vi "MotionProfileUpdateBuffers.vi"(3 "error in":errorcluster, 4 "RobotConfig":T1={"Motors"={"DriveRightPrimary"={"CAN Address"=3, "Invert"=FALSE, "InvertSensor"=FALSE, "Unit Conversion Factor"=0.0, "Brake Mode"=enum."Override to Brake", "Reverse Limt Switch Mode"=enum."Normally Closed", "Forward Limt Swith Mode"=enum."Normally Closed", "PWM Channel"=enum."Invalid", "Motor Controller Type"=enum."Talon SRX", "Peak Current (A)"=0, "Continuos Current (A)"=0, "Peak Duration (ms)"=0, "Current Limit Enable"=FALSE}, "DriveRightSecondary"={"CAN Address"=2, "Invert"=FALSE, "InvertSensor"=FALSE, "Unit Conversion Factor"=0.0, "Brake Mode"=enum."Override to Brake", "Reverse Limt Switch Mode"=enum."Normally Closed", "Forward Limt Swith Mode"=enum."Normally Closed", "PWM Channel"=enum."Invalid", "Motor Controller Type"=enum."Talon SRX", "Peak Current (A)"=0, "Continuos Current (A)"=0, "Peak Duration (ms)"=0, "Current Limit Enable"=FALSE}, "DriveLeftPrimary"={"CAN Address"=1, "Invert"=FALSE, "InvertSensor"=FALSE, "Unit Conversion Factor"=0.0, "Brake Mode"=enum."Override to Brake", "Reverse Limt Switch Mode"=enum."Normally Closed", "Forward Limt Swith Mode"=enum."Normally Closed", "PWM Channel"=enum."Invalid", "Motor Controller Type"=enum."Talon SRX", "Peak Current (A)"=0, "Continuos Current (A)"=0, "Peak Duration (ms)"=0, "Current Limit Enable"=FALSE}, "DriveLeftSecondary"={"CAN Address"=4, "Invert"=FALSE, "InvertSensor"=FALSE, "Unit Conversion Factor"=0.0, "Brake Mode"=enum."Override to Brake", "Reverse Limt Switch Mode"=enum."Normally Closed", "Forward Limt Swith Mode"=enum."Normally Closed", "PWM Channel"=enum."Invalid", "Motor Controller Type"=enum."Talon SRX", "Peak Current (A)"=0, "Continuos Current (A)"=0, "Peak Duration (ms)"=0, "Current Limit Enable"=FALSE}, "RearClimb"={"CAN Address"=8, "Invert"=FALSE, "InvertSensor"=FALSE, "Unit Conversion Factor"=0.0, "Brake Mode"=enum."Override to Brake", "Reverse Limt Switch Mode"=enum."Normally Closed", "Forward Limt Swith Mode"=enum."Normally Closed", "PWM Channel"=enum."Invalid", "Motor Controller Type"=enum."Talon SRX", "Peak Current (A)"=0, "Continuos Current (A)"=0, "Peak Duration (ms)"=0, "Current Limit Enable"=FALSE}, "Front Climb"={"CAN Address"=7, "Invert"=FALSE, "InvertSensor"=FALSE, "Unit Conversion Factor"=0.0, "Brake Mode"=enum."Override to Brake", "Reverse Limt Switch Mode"=enum."Normally Closed", "Forward Limt Swith Mode"=enum."Normally Closed", "PWM Channel"=enum."Invalid", "Motor Controller Type"=enum."Talon SRX", "Peak Current (A)"=0, "Continuos Current (A)"=0, "Peak Duration (ms)"=0, "Current Limit Enable"=FALSE}, "Climb Drive"={"CAN Address"=5, "Invert"=FALSE, "InvertSensor"=FALSE, "Unit Conversion Factor"=0.0, "Brake Mode"=enum."Override to Brake", "Reverse Limt Switch Mode"=enum."Normally Closed", "Forward Limt Swith Mode"=enum."Normally Closed", "PWM Channel"=enum."Invalid", "Motor Controller Type"=enum."Talon SRX", "Peak Current (A)"=0, "Continuos Current (A)"=0, "Peak Duration (ms)"=0, "Current Limit Enable"=FALSE}, "Shoulder1"={"CAN Address"=6, "Invert"=FALSE, "InvertSensor"=FALSE, "Unit Conversion Factor"=0.0, "Brake Mode"=enum."Override to Brake", "Reverse Limt Switch Mode"=enum."Normally Closed", "Forward Limt Swith Mode"=enum."Normally Closed", "PWM Channel"=enum."Invalid", "Motor Controller Type"=enum."Talon SRX", "Peak Current (A)"=0, "Continuos Current (A)"=0, "Peak Duration (ms)"=0, "Current Limit Enable"=FALSE}, "Shoulder2"={"CAN Address"=9, "Invert"=FALSE, "InvertSensor"=FALSE, "Unit Conversion Factor"=0.0, "Brake Mode"=enum."Override to Brake", "Reverse Limt Switch Mode"=enum."Normally Closed", "Forward Limt Swith Mode"=enum."Normally Closed", "PWM Channel"=enum."Invalid", "Motor Controller Type"=enum."Talon SRX", "Peak Current (A)"=0, "Continuos Current (A)"=0, "Peak Duration (ms)"=0, "Current Limit Enable"=FALSE}, "Wrist"={"CAN Address"=10, "Invert"=FALSE, "InvertSensor"=FALSE, "Unit Conversion Factor"=0.0, "Brake Mode"=enum."Override to Brake", "Reverse Limt Switch Mode"=enum."Disabled", "Forward Limt Swith Mode"=enum."Disabled", "PWM Channel"=enum."Invalid", "Motor Controller Type"=enum."Talon SRX", "Peak Current (A)"=0, "Continuos Current (A)"=0, "Peak Duration (ms)"=0, "Current Limit Enable"=FALSE}, "Extension"={"CAN Address"=11, "Invert"=FALSE, "InvertSensor"=FALSE, "Unit Conversion Factor"=0.0, "Brake Mode"=enum."Override to Brake", "Reverse Limt Switch Mode"=enum."Disabled", "Forward Limt Swith Mode"=enum."Disabled", "PWM Channel"=enum."Invalid", "Motor Controller Type"=enum."Talon SRX", "Peak Current (A)"=0, "Continuos Current (A)"=0, "Peak Duration (ms)"=0, "Current Limit Enable"=FALSE}, "Intake1"={"CAN Address"=0, "Invert"=FALSE, "InvertSensor"=FALSE, "Unit Conversion Factor"=1.0, "Brake Mode"=enum."Override to Brake", "Reverse Limt Switch Mode"=enum."Disabled", "Forward Limt Swith Mode"=enum."Normally Open", "PWM Channel"=enum."PWM 8", "Motor Controller Type"=enum."Talon SR", "Peak Current (A)"=0, "Continuos Current (A)"=0, "Peak Duration (ms)"=0, "Current Limit Enable"=FALSE}, "Intake2"={"CAN Address"=10, "Invert"=FALSE, "InvertSensor"=TRUE, "Unit Conversion Factor"=0.0, "Brake Mode"=enum."Override to Brake", "Reverse Limt Switch Mode"=enum."Normally Open", "Forward Limt Swith Mode"=enum."Normally Open", "PWM Channel"=enum."PWM 0", "Motor Controller Type"=enum."Disabled", "Peak Current (A)"=0, "Continuos Current (A)"=0, "Peak Duration (ms)"=0, "Current Limit Enable"=FALSE}}, "Sensors"={"IMU"={"Yaw Axis"=enum."Z", "SPI Bus"=enum."SPI MXP", "AHRS Algorithm"=enum."Complementary", "Calibration Time (s)"=3.0, "Calibrate On Open"=TRUE}}, "PID"={"FrontClimb"={"P"=0.0, "I"=0.0, "D"=0.0, "F"=0.0, "IZone"=0.0}, "RearClimb"={"P"=0.0, "I"=0.0, "D"=0.0, "F"=0.0, "IZone"=0.0}, "ArmShoulder"={"P"=0.0, "I"=0.0, "D"=0.0, "F"=0.0, "IZone"=0.0}, "ArmExtend"={"P"=0.0, "I"=0.0, "D"=0.0, "F"=0.0, "IZone"=0.0}, "ArmWrist"={"P"=0.0, "I"=0.0, "D"=0.0, "F"=0.0, "IZone"=0.0}}, "Solenoids"={" Shifter"={"SolenoidChannel"=enum."Solenoid 3", "Invert"=FALSE}, "Hatch Grip"={"SolenoidChannel"=enum."Solenoid 0", "Invert"=FALSE}, "Hatch Extend"={"SolenoidChannel"=enum."Solenoid 1", "Invert"=FALSE}, "Manipulator Slide"={"SolenoidChannel"=enum."Solenoid 2", "Invert"=FALSE}, "Hatch Floor Intake"={"SolenoidChannel"=enum."Solenoid 0", "Invert"=FALSE}}, "Enable Compressor"=TRUE, "MotionMagic"={"FrontClimb"={"CruiseVelocity"=0, "Acceleration"=0}, "RearClimb"={"CruiseVelocity"=0, "Acceleration"=0}}, "RobotDimensions"={"Length (in)"=0.0, "Shoulder Height (in)"=0.0, "Frame Height (in)"=0.0, "Arm Center to Front of Robot (in)"=0.0, "Arm Min Extension (in)"=0.0, "Arm Max Extension (in)"=0.0}, "Arm Home Position"={"Radius (in)"=0.0, "ShoulderAngle (rad)"=0.0, "WristAngle (rad)"=0.0}}, 5 "RobotMotors":T15={"DriveRightPrimary"={"DeviceStatus"={"status"=FALSE, "code"=0, "source"=""}, "Type"=enum."PWM", "PWM"={"PWM Channel"=enum."PWM 1", "DeadBand"={"Name"="", "maxPositivePwm"=0, "minPositivePwm"=0, "centerPwm"=0, "maxNegativePwm"=0, "minNegativePwm"=0, "angularRange"=0}}, "CAN"={"Device Number"=0, "SetOutput VI Ref"=variant(enum8{"Percent VBus", "Current", "Speed", "Position", "Voltage"} enum."Percent VBus"), "GetOutput VI Ref"=variant(refnum<k1> refnum), "Enable VI Ref"=variant(dbl 12.0), "Disable VI Ref"=variant(enum8{"Percent VBus", "Speed", "Position", "Slave", "Unchanged / Invalid", "Voltage Compensation", "Current", "Motion Profile"} enum."Percent VBus"), "Data"=variant}, "Invert"=FALSE, "DIO PWM"={"PWM \"Enable\" Channel"=enum."Invalid", "DIOChannel"=enum."Invalid", "PWM Rate"=0.0}}, "DriveRightSecondary"={"DeviceStatus"={"status"=FALSE, "code"=0, "source"=""}, "Type"=enum."PWM", "PWM"={"PWM Channel"=enum."PWM 1", "DeadBand"={"Name"="", "maxPositivePwm"=0, "minPositivePwm"=0, "centerPwm"=0, "maxNegativePwm"=0, "minNegativePwm"=0, "angularRange"=0}}, "CAN"={"Device Number"=0, "SetOutput VI Ref"=variant(enum8{"Percent VBus", "Current", "Speed", "Position", "Voltage"} enum."Percent VBus"), "GetOutput VI Ref"=variant(refnum<k1> refnum), "Enable VI Ref"=variant(dbl 12.0), "Disable VI Ref"=variant(enum8{"Percent VBus", "Speed", "Position", "Slave", "Unchanged / Invalid", "Voltage Compensation", "Current", "Motion Profile"} enum."Percent VBus"), "Data"=variant}, "Invert"=FALSE, "DIO PWM"={"PWM \"Enable\" Channel"=enum."Invalid", "DIOChannel"=enum."Invalid", "PWM Rate"=0.0}}, "DriveLeftPrimary"={"DeviceStatus"={"status"=FALSE, "code"=0, "source"=""}, "Type"=enum."PWM", "PWM"={"PWM Channel"=enum."PWM 1", "DeadBand"={"Name"="", "maxPositivePwm"=0, "minPositivePwm"=0, "centerPwm"=0, "maxNegativePwm"=0, "minNegativePwm"=0, "angularRange"=0}}, "CAN"={"Device Number"=0, "SetOutput VI Ref"=variant(enum8{"Percent VBus", "Current", "Speed", "Position", "Voltage"} enum."Percent VBus"), "GetOutput VI Ref"=variant(refnum<k1> refnum), "Enable VI Ref"=variant(dbl 12.0), "Disable VI Ref"=variant(enum8{"Percent VBus", "Speed", "Position", "Slave", "Unchanged / Invalid", "Voltage Compensation", "Current", "Motion Profile"} enum."Percent VBus"), "Data"=variant}, "Invert"=FALSE, "DIO PWM"={"PWM \"Enable\" Channel"=enum."Invalid", "DIOChannel"=enum."Invalid", "PWM Rate"=0.0}}, "DriveLeftSecondary"={"DeviceStatus"={"status"=FALSE, "code"=0, "source"=""}, "Type"=enum."PWM", "PWM"={"PWM Channel"=enum."PWM 1", "DeadBand"={"Name"="", "maxPositivePwm"=0, "minPositivePwm"=0, "centerPwm"=0, "maxNegativePwm"=0, "minNegativePwm"=0, "angularRange"=0}}, "CAN"={"Device Number"=0, "SetOutput VI Ref"=variant(enum8{"Percent VBus", "Current", "Speed", "Position", "Voltage"} enum."Percent VBus"), "GetOutput VI Ref"=variant(refnum<k1> refnum), "Enable VI Ref"=variant(dbl 12.0), "Disable VI Ref"=variant(enum8{"Percent VBus", "Speed", "Position", "Slave", "Unchanged / Invalid", "Voltage Compensation", "Current", "Motion Profile"} enum."Percent VBus"), "Data"=variant}, "Invert"=FALSE, "DIO PWM"={"PWM \"Enable\" Channel"=enum."Invalid", "DIOChannel"=enum."Invalid", "PWM Rate"=0.0}}, " RearClimb"={"DeviceStatus"={"status"=FALSE, "code"=0, "source"=""}, "Type"=enum."PWM", "PWM"={"PWM Channel"=enum."PWM 1", "DeadBand"={"Name"="", "maxPositivePwm"=0, "minPositivePwm"=0, "centerPwm"=0, "maxNegativePwm"=0, "minNegativePwm"=0, "angularRange"=0}}, "CAN"={"Device Number"=0, "SetOutput VI Ref"=variant(enum8{"Percent VBus", "Current", "Speed", "Position", "Voltage"} enum."Percent VBus"), "GetOutput VI Ref"=variant(refnum<k1> refnum), "Enable VI Ref"=variant(dbl 12.0), "Disable VI Ref"=variant(enum8{"Percent VBus", "Speed", "Position", "Slave", "Unchanged / Invalid", "Voltage Compensation", "Current", "Motion Profile"} enum."Percent VBus"), "Data"=variant}, "Invert"=FALSE, "DIO PWM"={"PWM \"Enable\" Channel"=enum."Invalid", "DIOChannel"=enum."Invalid", "PWM Rate"=0.0}}, "FrontClimb"={"DeviceStatus"={"status"=FALSE, "code"=0, "source"=""}, "Type"=enum."PWM", "PWM"={"PWM Channel"=enum."PWM 1", "DeadBand"={"Name"="", "maxPositivePwm"=0, "minPositivePwm"=0, "centerPwm"=0, "maxNegativePwm"=0, "minNegativePwm"=0, "angularRange"=0}}, "CAN"={"Device Number"=0, "SetOutput VI Ref"=variant(enum8{"Percent VBus", "Current", "Speed", "Position", "Voltage"} enum."Percent VBus"), "GetOutput VI Ref"=variant(refnum<k1> refnum), "Enable VI Ref"=variant(dbl 12.0), "Disable VI Ref"=variant(enum8{"Percent VBus", "Speed", "Position", "Slave", "Unchanged / Invalid", "Voltage Compensation", "Current", "Motion Profile"} enum."Percent VBus"), "Data"=variant}, "Invert"=FALSE, "DIO PWM"={"PWM \"Enable\" Channel"=enum."Invalid", "DIOChannel"=enum."Invalid", "PWM Rate"=0.0}}, "ClimbDrive"={"DeviceStatus"={"status"=FALSE, "code"=0, "source"=""}, "Type"=enum."PWM", "PWM"={"PWM Channel"=enum."PWM 1", "DeadBand"={"Name"="", "maxPositivePwm"=0, "minPositivePwm"=0, "centerPwm"=0, "maxNegativePwm"=0, "minNegativePwm"=0, "angularRange"=0}}, "CAN"={"Device Number"=0, "SetOutput VI Ref"=variant(enum8{"Percent VBus", "Current", "Speed", "Position", "Voltage"} enum."Percent VBus"), "GetOutput VI Ref"=variant(refnum<k1> refnum), "Enable VI Ref"=variant(dbl 12.0), "Disable VI Ref"=variant(enum8{"Percent VBus", "Speed", "Position", "Slave", "Unchanged / Invalid", "Voltage Compensation", "Current", "Motion Profile"} enum."Percent VBus"), "Data"=variant}, "Invert"=FALSE, "DIO PWM"={"PWM \"Enable\" Channel"=enum."Invalid", "DIOChannel"=enum."Invalid", "PWM Rate"=0.0}}, "Shoulder2"={"DeviceStatus"={"status"=FALSE, "code"=0, "source"=""}, "Type"=enum."PWM", "PWM"={"PWM Channel"=enum."PWM 1", "DeadBand"={"Name"="", "maxPositivePwm"=0, "minPositivePwm"=0, "centerPwm"=0, "maxNegativePwm"=0, "minNegativePwm"=0, "angularRange"=0}}, "CAN"={"Device Number"=0, "SetOutput VI Ref"=variant(enum8{"Percent VBus", "Current", "Speed", "Position", "Voltage"} enum."Percent VBus"), "GetOutput VI Ref"=variant(refnum<k1> refnum), "Enable VI Ref"=variant(dbl 12.0), "Disable VI Ref"=variant(enum8{"Percent VBus", "Speed", "Position", "Slave", "Unchanged / Invalid", "Voltage Compensation", "Current", "Motion Profile"} enum."Percent VBus"), "Data"=variant}, "Invert"=FALSE, "DIO PWM"={"PWM \"Enable\" Channel"=enum."Invalid", "DIOChannel"=enum."Invalid", "PWM Rate"=0.0}}, "Shoulder1 "={"DeviceStatus"={"status"=FALSE, "code"=0, "source"=""}, "Type"=enum."PWM", "PWM"={"PWM Channel"=enum."PWM 1", "DeadBand"={"Name"="", "maxPositivePwm"=0, "minPositivePwm"=0, "centerPwm"=0, "maxNegativePwm"=0, "minNegativePwm"=0, "angularRange"=0}}, "CAN"={"Device Number"=0, "SetOutput VI Ref"=variant(enum8{"Percent VBus", "Current", "Speed", "Position", "Voltage"} enum."Percent VBus"), "GetOutput VI Ref"=variant(refnum<k1> refnum), "Enable VI Ref"=variant(dbl 12.0), "Disable VI Ref"=variant(enum8{"Percent VBus", "Speed", "Position", "Slave", "Unchanged / Invalid", "Voltage Compensation", "Current", "Motion Profile"} enum."Percent VBus"), "Data"=variant}, "Invert"=FALSE, "DIO PWM"={"PWM \"Enable\" Channel"=enum."Invalid", "DIOChannel"=enum."Invalid", "PWM Rate"=0.0}}, "Wrist"={"DeviceStatus"={"status"=FALSE, "code"=0, "source"=""}, "Type"=enum."PWM", "PWM"={"PWM Channel"=enum."PWM 1", "DeadBand"={"Name"="", "maxPositivePwm"=0, "minPositivePwm"=0, "centerPwm"=0, "maxNegativePwm"=0, "minNegativePwm"=0, "angularRange"=0}}, "CAN"={"Device Number"=0, "SetOutput VI Ref"=variant(enum8{"Percent VBus", "Current", "Speed", "Position", "Voltage"} enum."Percent VBus"), "GetOutput VI Ref"=variant(refnum<k1> refnum), "Enable VI Ref"=variant(dbl 12.0), "Disable VI Ref"=variant(enum8{"Percent VBus", "Speed", "Position", "Slave", "Unchanged / Invalid", "Voltage Compensation", "Current", "Motion Profile"} enum."Percent VBus"), "Data"=variant}, "Invert"=FALSE, "DIO PWM"={"PWM \"Enable\" Channel"=enum."Invalid", "DIOChannel"=enum."Invalid", "PWM Rate"=0.0}}, "Extension"={"DeviceStatus"={"status"=FALSE, "code"=0, "source"=""}, "Type"=enum."PWM", "PWM"={"PWM Channel"=enum."PWM 1", "DeadBand"={"Name"="", "maxPositivePwm"=0, "minPositivePwm"=0, "centerPwm"=0, "maxNegativePwm"=0, "minNegativePwm"=0, "angularRange"=0}}, "CAN"={"Device Number"=0, "SetOutput VI Ref"=variant(enum8{"Percent VBus", "Current", "Speed", "Position", "Voltage"} enum."Percent VBus"), "GetOutput VI Ref"=variant(refnum<k1> refnum), "Enable VI Ref"=variant(dbl 12.0), "Disable VI Ref"=variant(enum8{"Percent VBus", "Speed", "Position", "Slave", "Unchanged / Invalid", "Voltage Compensation", "Current", "Motion Profile"} enum."Percent VBus"), "Data"=variant}, "Invert"=FALSE, "DIO PWM"={"PWM \"Enable\" Channel"=enum."Invalid", "DIOChannel"=enum."Invalid", "PWM Rate"=0.0}}, "Intake1"={"DeviceStatus"={"status"=FALSE, "code"=0, "source"=""}, "Type"=enum."PWM", "PWM"={"PWM Channel"=enum."PWM 1", "DeadBand"={"Name"="", "maxPositivePwm"=0, "minPositivePwm"=0, "centerPwm"=0, "maxNegativePwm"=0, "minNegativePwm"=0, "angularRange"=0}}, "CAN"={"Device Number"=0, "SetOutput VI Ref"=variant(enum8{"Percent VBus", "Current", "Speed", "Position", "Voltage"} enum."Percent VBus"), "GetOutput VI Ref"=variant(refnum<k1> refnum), "Enable VI Ref"=variant(dbl 12.0), "Disable VI Ref"=variant(enum8{"Percent VBus", "Speed", "Position", "Slave", "Unchanged / Invalid", "Voltage Compensation", "Current", "Motion Profile"} enum."Percent VBus"), "Data"=variant}, "Invert"=FALSE, "DIO PWM"={"PWM \"Enable\" Channel"=enum."Invalid", "DIOChannel"=enum."Invalid", "PWM Rate"=0.0}}, "Intake2"={"DeviceStatus"={"status"=FALSE, "code"=0, "source"=""}, "Type"=enum."PWM", "PWM"={"PWM Channel"=enum."PWM 1", "DeadBand"={"Name"="", "maxPositivePwm"=0, "minPositivePwm"=0, "centerPwm"=0, "maxNegativePwm"=0, "minNegativePwm"=0, "angularRange"=0}}, "CAN"={"Device Number"=0, "SetOutput VI Ref"=variant(enum8{"Percent VBus", "Current", "Speed", "Position", "Voltage"} enum."Percent VBus"), "GetOutput VI Ref"=variant(refnum<k1> refnum), "Enable VI Ref"=variant(dbl 12.0), "Disable VI Ref"=variant(enum8{"Percent VBus", "Speed", "Position", "Slave", "Unchanged / Invalid", "Voltage Compensation", "Current", "Motion Profile"} enum."Percent VBus"), "Data"=variant}, "Invert"=FALSE, "DIO PWM"={"PWM \"Enable\" Channel"=enum."Invalid", "DIOChannel"=enum."Invalid", "PWM Rate"=0.0}}}) -> (0 "error out":errorcluster, 1 "RobotConfigOut":T1={"Motors"={"DriveRightPrimary"={"CAN Address"=3, "Invert"=FALSE, "InvertSensor"=FALSE, "Unit Conversion Factor"=0.0, "Brake Mode"=enum."Override to Brake", "Reverse Limt Switch Mode"=enum."Normally Closed", "Forward Limt Swith Mode"=enum."Normally Closed", "PWM Channel"=enum."Invalid", "Motor Controller Type"=enum."Talon SRX", "Peak Current (A)"=0, "Continuos Current (A)"=0, "Peak Duration (ms)"=0, "Current Limit Enable"=FALSE}, "DriveRightSecondary"={"CAN Address"=2, "Invert"=FALSE, "InvertSensor"=FALSE, "Unit Conversion Factor"=0.0, "Brake Mode"=enum."Override to Brake", "Reverse Limt Switch Mode"=enum."Normally Closed", "Forward Limt Swith Mode"=enum."Normally Closed", "PWM Channel"=enum."Invalid", "Motor Controller Type"=enum."Talon SRX", "Peak Current (A)"=0, "Continuos Current (A)"=0, "Peak Duration (ms)"=0, "Current Limit Enable"=FALSE}, "DriveLeftPrimary"={"CAN Address"=1, "Invert"=FALSE, "InvertSensor"=FALSE, "Unit Conversion Factor"=0.0, "Brake Mode"=enum."Override to Brake", "Reverse Limt Switch Mode"=enum."Normally Closed", "Forward Limt Swith Mode"=enum."Normally Closed", "PWM Channel"=enum."Invalid", "Motor Controller Type"=enum."Talon SRX", "Peak Current (A)"=0, "Continuos Current (A)"=0, "Peak Duration (ms)"=0, "Current Limit Enable"=FALSE}, "DriveLeftSecondary"={"CAN Address"=4, "Invert"=FALSE, "InvertSensor"=FALSE, "Unit Conversion Factor"=0.0, "Brake Mode"=enum."Override to Brake", "Reverse Limt Switch Mode"=enum."Normally Closed", "Forward Limt Swith Mode"=enum."Normally Closed", "PWM Channel"=enum."Invalid", "Motor Controller Type"=enum."Talon SRX", "Peak Current (A)"=0, "Continuos Current (A)"=0, "Peak Duration (ms)"=0, "Current Limit Enable"=FALSE}, "RearClimb"={"CAN Address"=8, "Invert"=FALSE, "InvertSensor"=FALSE, "Unit Conversion Factor"=0.0, "Brake Mode"=enum."Override to Brake", "Reverse Limt Switch Mode"=enum."Normally Closed", "Forward Limt Swith Mode"=enum."Normally Closed", "PWM Channel"=enum."Invalid", "Motor Controller Type"=enum."Talon SRX", "Peak Current (A)"=0, "Continuos Current (A)"=0, "Peak Duration (ms)"=0, "Current Limit Enable"=FALSE}, "Front Climb"={"CAN Address"=7, "Invert"=FALSE, "InvertSensor"=FALSE, "Unit Conversion Factor"=0.0, "Brake Mode"=enum."Override to Brake", "Reverse Limt Switch Mode"=enum."Normally Closed", "Forward Limt Swith Mode"=enum."Normally Closed", "PWM Channel"=enum."Invalid", "Motor Controller Type"=enum."Talon SRX", "Peak Current (A)"=0, "Continuos Current (A)"=0, "Peak Duration (ms)"=0, "Current Limit Enable"=FALSE}, "Climb Drive"={"CAN Address"=5, "Invert"=FALSE, "InvertSensor"=FALSE, "Unit Conversion Factor"=0.0, "Brake Mode"=enum."Override to Brake", "Reverse Limt Switch Mode"=enum."Normally Closed", "Forward Limt Swith Mode"=enum."Normally Closed", "PWM Channel"=enum."Invalid", "Motor Controller Type"=enum."Talon SRX", "Peak Current (A)"=0, "Continuos Current (A)"=0, "Peak Duration (ms)"=0, "Current Limit Enable"=FALSE}, "Shoulder1"={"CAN Address"=6, "Invert"=FALSE, "InvertSensor"=FALSE, "Unit Conversion Factor"=0.0, "Brake Mode"=enum."Override to Brake", "Reverse Limt Switch Mode"=enum."Normally Closed", "Forward Limt Swith Mode"=enum."Normally Closed", "PWM Channel"=enum."Invalid", "Motor Controller Type"=enum."Talon SRX", "Peak Current (A)"=0, "Continuos Current (A)"=0, "Peak Duration (ms)"=0, "Current Limit Enable"=FALSE}, "Shoulder2"={"CAN Address"=9, "Invert"=FALSE, "InvertSensor"=FALSE, "Unit Conversion Factor"=0.0, "Brake Mode"=enum."Override to Brake", "Reverse Limt Switch Mode"=enum."Normally Closed", "Forward Limt Swith Mode"=enum."Normally Closed", "PWM Channel"=enum."Invalid", "Motor Controller Type"=enum."Talon SRX", "Peak Current (A)"=0, "Continuos Current (A)"=0, "Peak Duration (ms)"=0, "Current Limit Enable"=FALSE}, "Wrist"={"CAN Address"=10, "Invert"=FALSE, "InvertSensor"=FALSE, "Unit Conversion Factor"=0.0, "Brake Mode"=enum."Override to Brake", "Reverse Limt Switch Mode"=enum."Disabled", "Forward Limt Swith Mode"=enum."Disabled", "PWM Channel"=enum."Invalid", "Motor Controller Type"=enum."Talon SRX", "Peak Current (A)"=0, "Continuos Current (A)"=0, "Peak Duration (ms)"=0, "Current Limit Enable"=FALSE}, "Extension"={"CAN Address"=11, "Invert"=FALSE, "InvertSensor"=FALSE, "Unit Conversion Factor"=0.0, "Brake Mode"=enum."Override to Brake", "Reverse Limt Switch Mode"=enum."Disabled", "Forward Limt Swith Mode"=enum."Disabled", "PWM Channel"=enum."Invalid", "Motor Controller Type"=enum."Talon SRX", "Peak Current (A)"=0, "Continuos Current (A)"=0, "Peak Duration (ms)"=0, "Current Limit Enable"=FALSE}, "Intake1"={"CAN Address"=0, "Invert"=FALSE, "InvertSensor"=FALSE, "Unit Conversion Factor"=1.0, "Brake Mode"=enum."Override to Brake", "Reverse Limt Switch Mode"=enum."Disabled", "Forward Limt Swith Mode"=enum."Normally Open", "PWM Channel"=enum."PWM 8", "Motor Controller Type"=enum."Talon SR", "Peak Current (A)"=0, "Continuos Current (A)"=0, "Peak Duration (ms)"=0, "Current Limit Enable"=FALSE}, "Intake2"={"CAN Address"=10, "Invert"=FALSE, "InvertSensor"=TRUE, "Unit Conversion Factor"=0.0, "Brake Mode"=enum."Override to Brake", "Reverse Limt Switch Mode"=enum."Normally Open", "Forward Limt Swith Mode"=enum."Normally Open", "PWM Channel"=enum."PWM 0", "Motor Controller Type"=enum."Disabled", "Peak Current (A)"=0, "Continuos Current (A)"=0, "Peak Duration (ms)"=0, "Current Limit Enable"=FALSE}}, "Sensors"={"IMU"={"Yaw Axis"=enum."Z", "SPI Bus"=enum."SPI MXP", "AHRS Algorithm"=enum."Complementary", "Calibration Time (s)"=3.0, "Calibrate On Open"=TRUE}}, "PID"={"FrontClimb"={"P"=0.0, "I"=0.0, "D"=0.0, "F"=0.0, "IZone"=0.0}, "RearClimb"={"P"=0.0, "I"=0.0, "D"=0.0, "F"=0.0, "IZone"=0.0}, "ArmShoulder"={"P"=0.0, "I"=0.0, "D"=0.0, "F"=0.0, "IZone"=0.0}, "ArmExtend"={"P"=0.0, "I"=0.0, "D"=0.0, "F"=0.0, "IZone"=0.0}, "ArmWrist"={"P"=0.0, "I"=0.0, "D"=0.0, "F"=0.0, "IZone"=0.0}}, "Solenoids"={" Shifter"={"SolenoidChannel"=enum."Solenoid 3", "Invert"=FALSE}, "Hatch Grip"={"SolenoidChannel"=enum."Solenoid 0", "Invert"=FALSE}, "Hatch Extend"={"SolenoidChannel"=enum."Solenoid 1", "Invert"=FALSE}, "Manipulator Slide"={"SolenoidChannel"=enum."Solenoid 2", "Invert"=FALSE}, "Hatch Floor Intake"={"SolenoidChannel"=enum."Solenoid 0", "Invert"=FALSE}}, "Enable Compressor"=TRUE, "MotionMagic"={"FrontClimb"={"CruiseVelocity"=0, "Acceleration"=0}, "RearClimb"={"CruiseVelocity"=0, "Acceleration"=0}}, "RobotDimensions"={"Length (in)"=0.0, "Shoulder Height (in)"=0.0, "Frame Height (in)"=0.0, "Arm Center to Front of Robot (in)"=0.0, "Arm Min Extension (in)"=0.0, "Arm Max Extension (in)"=0.0}, "Arm Home Position"={"Radius (in)"=0.0, "ShoulderAngle (rad)"=0.0, "WristAngle (rad)"=0.0}}, 2 "RobotMotorsOut":T15={"DriveRightPrimary"={"DeviceStatus"={"status"=FALSE, "code"=0, "source"=""}, "Type"=enum."PWM", "PWM"={"PWM Channel"=enum."PWM 1", "DeadBand"={"Name"="", "maxPositivePwm"=0, "minPositivePwm"=0, "centerPwm"=0, "maxNegativePwm"=0, "minNegativePwm"=0, "angularRange"=0}}, "CAN"={"Device Number"=0, "SetOutput VI Ref"=variant(enum8{"Percent VBus", "Current", "Speed", "Position", "Voltage"} enum."Percent VBus"), "GetOutput VI Ref"=variant(refnum<k1> refnum), "Enable VI Ref"=variant(dbl 12.0), "Disable VI Ref"=variant(enum8{"Percent VBus", "Speed", "Position", "Slave", "Unchanged / Invalid", "Voltage Compensation", "Current", "Motion Profile"} enum."Percent VBus"), "Data"=variant}, "Invert"=FALSE, "DIO PWM"={"PWM \"Enable\" Channel"=enum."Invalid", "DIOChannel"=enum."Invalid", "PWM Rate"=0.0}}, "DriveRightSecondary"={"DeviceStatus"={"status"=FALSE, "code"=0, "source"=""}, "Type"=enum."PWM", "PWM"={"PWM Channel"=enum."PWM 1", "DeadBand"={"Name"="", "maxPositivePwm"=0, "minPositivePwm"=0, "centerPwm"=0, "maxNegativePwm"=0, "minNegativePwm"=0, "angularRange"=0}}, "CAN"={"Device Number"=0, "SetOutput VI Ref"=variant(enum8{"Percent VBus", "Current", "Speed", "Position", "Voltage"} enum."Percent VBus"), "GetOutput VI Ref"=variant(refnum<k1> refnum), "Enable VI Ref"=variant(dbl 12.0), "Disable VI Ref"=variant(enum8{"Percent VBus", "Speed", "Position", "Slave", "Unchanged / Invalid", "Voltage Compensation", "Current", "Motion Profile"} enum."Percent VBus"), "Data"=variant}, "Invert"=FALSE, "DIO PWM"={"PWM \"Enable\" Channel"=enum."Invalid", "DIOChannel"=enum."Invalid", "PWM Rate"=0.0}}, "DriveLeftPrimary"={"DeviceStatus"={"status"=FALSE, "code"=0, "source"=""}, "Type"=enum."PWM", "PWM"={"PWM Channel"=enum."PWM 1", "DeadBand"={"Name"="", "maxPositivePwm"=0, "minPositivePwm"=0, "centerPwm"=0, "maxNegativePwm"=0, "minNegativePwm"=0, "angularRange"=0}}, "CAN"={"Device Number"=0, "SetOutput VI Ref"=variant(enum8{"Percent VBus", "Current", "Speed", "Position", "Voltage"} enum."Percent VBus"), "GetOutput VI Ref"=variant(refnum<k1> refnum), "Enable VI Ref"=variant(dbl 12.0), "Disable VI Ref"=variant(enum8{"Percent VBus", "Speed", "Position", "Slave", "Unchanged / Invalid", "Voltage Compensation", "Current", "Motion Profile"} enum."Percent VBus"), "Data"=variant}, "Invert"=FALSE, "DIO PWM"={"PWM \"Enable\" Channel"=enum."Invalid", "DIOChannel"=enum."Invalid", "PWM Rate"=0.0}}, "DriveLeftSecondary"={"DeviceStatus"={"status"=FALSE, "code"=0, "source"=""}, "Type"=enum."PWM", "PWM"={"PWM Channel"=enum."PWM 1", "DeadBand"={"Name"="", "maxPositivePwm"=0, "minPositivePwm"=0, "centerPwm"=0, "maxNegativePwm"=0, "minNegativePwm"=0, "angularRange"=0}}, "CAN"={"Device Number"=0, "SetOutput VI Ref"=variant(enum8{"Percent VBus", "Current", "Speed", "Position", "Voltage"} enum."Percent VBus"), "GetOutput VI Ref"=variant(refnum<k1> refnum), "Enable VI Ref"=variant(dbl 12.0), "Disable VI Ref"=variant(enum8{"Percent VBus", "Speed", "Position", "Slave", "Unchanged / Invalid", "Voltage Compensation", "Current", "Motion Profile"} enum."Percent VBus"), "Data"=variant}, "Invert"=FALSE, "DIO PWM"={"PWM \"Enable\" Channel"=enum."Invalid", "DIOChannel"=enum."Invalid", "PWM Rate"=0.0}}, " RearClimb"={"DeviceStatus"={"status"=FALSE, "code"=0, "source"=""}, "Type"=enum."PWM", "PWM"={"PWM Channel"=enum."PWM 1", "DeadBand"={"Name"="", "maxPositivePwm"=0, "minPositivePwm"=0, "centerPwm"=0, "maxNegativePwm"=0, "minNegativePwm"=0, "angularRange"=0}}, "CAN"={"Device Number"=0, "SetOutput VI Ref"=variant(enum8{"Percent VBus", "Current", "Speed", "Position", "Voltage"} enum."Percent VBus"), "GetOutput VI Ref"=variant(refnum<k1> refnum), "Enable VI Ref"=variant(dbl 12.0), "Disable VI Ref"=variant(enum8{"Percent VBus", "Speed", "Position", "Slave", "Unchanged / Invalid", "Voltage Compensation", "Current", "Motion Profile"} enum."Percent VBus"), "Data"=variant}, "Invert"=FALSE, "DIO PWM"={"PWM \"Enable\" Channel"=enum."Invalid", "DIOChannel"=enum."Invalid", "PWM Rate"=0.0}}, "FrontClimb"={"DeviceStatus"={"status"=FALSE, "code"=0, "source"=""}, "Type"=enum."PWM", "PWM"={"PWM Channel"=enum."PWM 1", "DeadBand"={"Name"="", "maxPositivePwm"=0, "minPositivePwm"=0, "centerPwm"=0, "maxNegativePwm"=0, "minNegativePwm"=0, "angularRange"=0}}, "CAN"={"Device Number"=0, "SetOutput VI Ref"=variant(enum8{"Percent VBus", "Current", "Speed", "Position", "Voltage"} enum."Percent VBus"), "GetOutput VI Ref"=variant(refnum<k1> refnum), "Enable VI Ref"=variant(dbl 12.0), "Disable VI Ref"=variant(enum8{"Percent VBus", "Speed", "Position", "Slave", "Unchanged / Invalid", "Voltage Compensation", "Current", "Motion Profile"} enum."Percent VBus"), "Data"=variant}, "Invert"=FALSE, "DIO PWM"={"PWM \"Enable\" Channel"=enum."Invalid", "DIOChannel"=enum."Invalid", "PWM Rate"=0.0}}, "ClimbDrive"={"DeviceStatus"={"status"=FALSE, "code"=0, "source"=""}, "Type"=enum."PWM", "PWM"={"PWM Channel"=enum."PWM 1", "DeadBand"={"Name"="", "maxPositivePwm"=0, "minPositivePwm"=0, "centerPwm"=0, "maxNegativePwm"=0, "minNegativePwm"=0, "angularRange"=0}}, "CAN"={"Device Number"=0, "SetOutput VI Ref"=variant(enum8{"Percent VBus", "Current", "Speed", "Position", "Voltage"} enum."Percent VBus"), "GetOutput VI Ref"=variant(refnum<k1> refnum), "Enable VI Ref"=variant(dbl 12.0), "Disable VI Ref"=variant(enum8{"Percent VBus", "Speed", "Position", "Slave", "Unchanged / Invalid", "Voltage Compensation", "Current", "Motion Profile"} enum."Percent VBus"), "Data"=variant}, "Invert"=FALSE, "DIO PWM"={"PWM \"Enable\" Channel"=enum."Invalid", "DIOChannel"=enum."Invalid", "PWM Rate"=0.0}}, "Shoulder2"={"DeviceStatus"={"status"=FALSE, "code"=0, "source"=""}, "Type"=enum."PWM", "PWM"={"PWM Channel"=enum."PWM 1", "DeadBand"={"Name"="", "maxPositivePwm"=0, "minPositivePwm"=0, "centerPwm"=0, "maxNegativePwm"=0, "minNegativePwm"=0, "angularRange"=0}}, "CAN"={"Device Number"=0, "SetOutput VI Ref"=variant(enum8{"Percent VBus", "Current", "Speed", "Position", "Voltage"} enum."Percent VBus"), "GetOutput VI Ref"=variant(refnum<k1> refnum), "Enable VI Ref"=variant(dbl 12.0), "Disable VI Ref"=variant(enum8{"Percent VBus", "Speed", "Position", "Slave", "Unchanged / Invalid", "Voltage Compensation", "Current", "Motion Profile"} enum."Percent VBus"), "Data"=variant}, "Invert"=FALSE, "DIO PWM"={"PWM \"Enable\" Channel"=enum."Invalid", "DIOChannel"=enum."Invalid", "PWM Rate"=0.0}}, "Shoulder1 "={"DeviceStatus"={"status"=FALSE, "code"=0, "source"=""}, "Type"=enum."PWM", "PWM"={"PWM Channel"=enum."PWM 1", "DeadBand"={"Name"="", "maxPositivePwm"=0, "minPositivePwm"=0, "centerPwm"=0, "maxNegativePwm"=0, "minNegativePwm"=0, "angularRange"=0}}, "CAN"={"Device Number"=0, "SetOutput VI Ref"=variant(enum8{"Percent VBus", "Current", "Speed", "Position", "Voltage"} enum."Percent VBus"), "GetOutput VI Ref"=variant(refnum<k1> refnum), "Enable VI Ref"=variant(dbl 12.0), "Disable VI Ref"=variant(enum8{"Percent VBus", "Speed", "Position", "Slave", "Unchanged / Invalid", "Voltage Compensation", "Current", "Motion Profile"} enum."Percent VBus"), "Data"=variant}, "Invert"=FALSE, "DIO PWM"={"PWM \"Enable\" Channel"=enum."Invalid", "DIOChannel"=enum."Invalid", "PWM Rate"=0.0}}, "Wrist"={"DeviceStatus"={"status"=FALSE, "code"=0, "source"=""}, "Type"=enum."PWM", "PWM"={"PWM Channel"=enum."PWM 1", "DeadBand"={"Name"="", "maxPositivePwm"=0, "minPositivePwm"=0, "centerPwm"=0, "maxNegativePwm"=0, "minNegativePwm"=0, "angularRange"=0}}, "CAN"={"Device Number"=0, "SetOutput VI Ref"=variant(enum8{"Percent VBus", "Current", "Speed", "Position", "Voltage"} enum."Percent VBus"), "GetOutput VI Ref"=variant(refnum<k1> refnum), "Enable VI Ref"=variant(dbl 12.0), "Disable VI Ref"=variant(enum8{"Percent VBus", "Speed", "Position", "Slave", "Unchanged / Invalid", "Voltage Compensation", "Current", "Motion Profile"} enum."Percent VBus"), "Data"=variant}, "Invert"=FALSE, "DIO PWM"={"PWM \"Enable\" Channel"=enum."Invalid", "DIOChannel"=enum."Invalid", "PWM Rate"=0.0}}, "Extension"={"DeviceStatus"={"status"=FALSE, "code"=0, "source"=""}, "Type"=enum."PWM", "PWM"={"PWM Channel"=enum."PWM 1", "DeadBand"={"Name"="", "maxPositivePwm"=0, "minPositivePwm"=0, "centerPwm"=0, "maxNegativePwm"=0, "minNegativePwm"=0, "angularRange"=0}}, "CAN"={"Device Number"=0, "SetOutput VI Ref"=variant(enum8{"Percent VBus", "Current", "Speed", "Position", "Voltage"} enum."Percent VBus"), "GetOutput VI Ref"=variant(refnum<k1> refnum), "Enable VI Ref"=variant(dbl 12.0), "Disable VI Ref"=variant(enum8{"Percent VBus", "Speed", "Position", "Slave", "Unchanged / Invalid", "Voltage Compensation", "Current", "Motion Profile"} enum."Percent VBus"), "Data"=variant}, "Invert"=FALSE, "DIO PWM"={"PWM \"Enable\" Channel"=enum."Invalid", "DIOChannel"=enum."Invalid", "PWM Rate"=0.0}}, "Intake1"={"DeviceStatus"={"status"=FALSE, "code"=0, "source"=""}, "Type"=enum."PWM", "PWM"={"PWM Channel"=enum."PWM 1", "DeadBand"={"Name"="", "maxPositivePwm"=0, "minPositivePwm"=0, "centerPwm"=0, "maxNegativePwm"=0, "minNegativePwm"=0, "angularRange"=0}}, "CAN"={"Device Number"=0, "SetOutput VI Ref"=variant(enum8{"Percent VBus", "Current", "Speed", "Position", "Voltage"} enum."Percent VBus"), "GetOutput VI Ref"=variant(refnum<k1> refnum), "Enable VI Ref"=variant(dbl 12.0), "Disable VI Ref"=variant(enum8{"Percent VBus", "Speed", "Position", "Slave", "Unchanged / Invalid", "Voltage Compensation", "Current", "Motion Profile"} enum."Percent VBus"), "Data"=variant}, "Invert"=FALSE, "DIO PWM"={"PWM \"Enable\" Channel"=enum."Invalid", "DIOChannel"=enum."Invalid", "PWM Rate"=0.0}}, "Intake2"={"DeviceStatus"={"status"=FALSE, "code"=0, "source"=""}, "Type"=enum."PWM", "PWM"={"PWM Channel"=enum."PWM 1", "DeadBand"={"Name"="", "maxPositivePwm"=0, "minPositivePwm"=0, "centerPwm"=0, "maxNegativePwm"=0, "minNegativePwm"=0, "angularRange"=0}}, "CAN"={"Device Number"=0, "SetOutput VI Ref"=variant(enum8{"Percent VBus", "Current", "Speed", "Position", "Voltage"} enum."Percent VBus"), "GetOutput VI Ref"=variant(refnum<k1> refnum), "Enable VI Ref"=variant(dbl 12.0), "Disable VI Ref"=variant(enum8{"Percent VBus", "Speed", "Position", "Slave", "Unchanged / Invalid", "Voltage Compensation", "Current", "Motion Profile"} enum."Percent VBus"), "Data"=variant}, "Invert"=FALSE, "DIO PWM"={"PWM \"Enable\" Channel"=enum."Invalid", "DIOChannel"=enum."Invalid", "PWM Rate"=0.0}}})   [LabVIEW 2018]
uses:
  TypeDefs/RobotComponents/RobotMotors.ctl
  <vilib>/Rock Robotics/WPI/MotorControl/WPI_MotorControlDeviceRef.ctl
  <vilib>/Rock Robotics/WPI/MotorControl/WPI_MotorControlType.ctl
  <vilib>/Rock Robotics/SystemInterfaces/DIO/FPGA_DIOPWMChannel.ctl
  <vilib>/Rock Robotics/WPI/PWM/WPI_PWMDeadband.ctl
  <vilib>/Rock Robotics/SystemInterfaces/DIO/FPGA_DIOChannel.ctl
  TypeDefs/ConfigComponents/Config_Robot.ctl
  ArgosLib/Config/ConfigComponents/TypeDefs/Config_Motor.ctl
  <vilib>/Rock Robotics/WPI/ThirdParty/Phoenix-LabVIEW/Motor Controller/Controls/CTRE_Phoenix_MotorControl_NeutralMode.ctl
  <vilib>/Rock Robotics/WPI/ThirdParty/Phoenix-LabVIEW/Motor Controller/Controls/CTRE_Phoenix_MotorControl_LimitSwitchNormal.ctl
  ArgosLib/Config/ConfigComponents/TypeDefs/Config_MotorCtrlType.ctl
  ArgosLib/Config/ConfigComponents/TypeDefs/Config_IMU.ctl
  <vilib>/Rock Robotics/SystemInterfaces/spilib/spi_bus.ctl
  ArgosLib/Config/ConfigComponents/TypeDefs/Config_PIDParams.ctl
  ArgosLib/Config/ConfigComponents/TypeDefs/Config_SingleSolenoid.ctl
  <vilib>/Rock Robotics/WPI/Solenoid/WPI_SolenoidChannel.ctl
  ArgosLib/Config/ConfigComponents/TypeDefs/Config_MotionMagicParams.ctl
  TypeDefs/ConfigComponents/Config_Dimensions.ctl
  Implements/Arm/TypeDefs/ArmCoordinate.ctl
  Global_Var-RefNum/MotionProfileControlData.vi
  ArgosLib/ArgosLib.lvlib
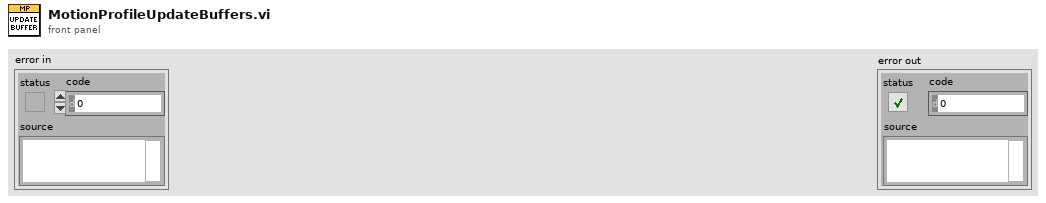
[diagram p1: front panel]
types:
  T1 = typedef "Config_Robot.ctl" = cluster{"Motors":cluster{"DriveRightPrimary":T2, "DriveRightSecondary":T2, "DriveLeftPrimary":T2, "DriveLeftSecondary":T2, "RearClimb":T2, "Front Climb":T2, "Climb Drive":T2, "Shoulder1":T2, "Shoulder2":T2, "Wrist":T2, "Extension":T2, "Intake1":T2, "Intake2":T2}, "Sensors":cluster{"IMU":T7}, "PID":cluster{"FrontClimb":T9, "RearClimb":T9, "ArmShoulder":T9, "ArmExtend":T9, "ArmWrist":T9}, "Solenoids":cluster{" Shifter":T10, "Hatch Grip":T10, "Hatch Extend":T10, "Manipulator Slide":T10, "Hatch Floor Intake":T10}, "Enable Compressor":bool, "MotionMagic":cluster{"FrontClimb":T12, "RearClimb":T12}, "RobotDimensions":T13, "Arm Home Position":T14}
  T2 = typedef "ArgosLib.lvlib/Config_Motor.ctl" = cluster{"CAN Address":u8, "Invert":bool, "InvertSensor":bool, "Unit Conversion Factor":dbl, "Brake Mode":T3, "Reverse Limt Switch Mode":T4, "Forward Limt Swith Mode":T4, "PWM Channel":T5, "Motor Controller Type":T6, "Peak Current (A)":i32, "Continuos Current (A)":i32, "Peak Duration (ms)":i32, "Current Limit Enable":bool}
  T3 = typedef "CTRE_Phoenix_MotorControl_NeutralMode.ctl" = enum8{"EEPROMSetting", "Override to Coast", "Override to Brake"}
  T4 = typedef "CTRE_Phoenix_MotorControl_LimitSwitchNormal.ctl" = enum16{"Normally Open", "Normally Closed", "Disabled"}
  T5 = typedef "FPGA_DIOPWMChannel.ctl" = enum8{"PWM 0", "PWM 1", "PWM 2", "PWM 3", "PWM 4", "PWM 5", "PWM 6", "PWM 7", "PWM 8", "PWM 9", "PWM MXP 0", "PWM MXP 1", "PWM MXP 2", "PWM MXP 3", "PWM MXP 4", "PWM MXP 5", "PWM MXP 6", "PWM MXP 7", "PWM MXP 8", "PWM MXP 9", "Invalid"}
  T6 = typedef "ArgosLib.lvlib/Config_MotorCtrlType.ctl" = enum16{"Disabled", "Talon SRX", "Talon SR"}
  T7 = typedef "ArgosLib.lvlib/Config_IMU.ctl" = cluster{"Yaw Axis":enum16{"X", "Y", "Z"}, "SPI Bus":T8, "AHRS Algorithm":enum16{"Complementary", "Madgwick"}, "Calibration Time (s)":dbl, "Calibrate On Open":bool}
  T8 = typedef "spi_bus.ctl" = enum16{"SPI On-Board, CS0", "SPI On-Board, CS1", "SPI On-Board, CS2", "SPI On-Board, CS3", "SPI MXP", "Invalid"}
  T9 = typedef "ArgosLib.lvlib/Config_PIDParams.ctl" = cluster{"P":dbl, "I":dbl, "D":dbl, "F":dbl, "IZone":dbl}
  T10 = typedef "ArgosLib.lvlib/Config_SingleSolenoid.ctl" = cluster{"SolenoidChannel":T11, "Invert":bool}
  T11 = typedef "WPI_SolenoidChannel.ctl" = enum8{"Solenoid 0", "Solenoid 1", "Solenoid 2", "Solenoid 3", "Solenoid 4", "Solenoid 5", "Solenoid 6", "Solenoid 7", "Invalid"}
  T12 = typedef "Config_MotionMagicParams.ctl" = cluster{"CruiseVelocity":i32, "Acceleration":i32}
  T13 = typedef "Config_Dimensions.ctl" = cluster{"Length (in)":dbl, "Shoulder Height (in)":dbl, "Frame Height (in)":dbl, "Arm Center to Front of Robot (in)":dbl, "Arm Min Extension (in)":dbl, "Arm Max Extension (in)":dbl}
  T14 = typedef "ArmCoordinate.ctl" = cluster{"Radius (in)":dbl, "ShoulderAngle (rad)":dbl, "WristAngle (rad)":dbl}
  T15 = typedef "RobotMotors.ctl" = cluster{"DriveRightPrimary":T16, "DriveRightSecondary":T16, "DriveLeftPrimary":T16, "DriveLeftSecondary":T16, " RearClimb":T16, "FrontClimb":T16, "ClimbDrive":T16, "Shoulder2":T16, "Shoulder1 ":T16, "Wrist":T16, "Extension":T16, "Intake1":T16, "Intake2":T16}
  T16 = typedef "WPI_MotorControlDeviceRef.ctl" = cluster{"DeviceStatus":errorcluster, "Type":T17, "PWM":cluster{"PWM Channel":T5, "DeadBand":T18}, "CAN":cluster{"Device Number":u8, "SetOutput VI Ref":variant, "GetOutput VI Ref":variant, "Enable VI Ref":variant, "Disable VI Ref":variant, "Data":variant}, "Invert":bool, "DIO PWM":cluster{"PWM \"Enable\" Channel":T5, "DIOChannel":T19, "PWM Rate":dbl}}
  T17 = typedef "WPI_MotorControlType.ctl" = enum16{"PWM", "CAN", "DIO PWM"}
  T18 = typedef "WPI_PWMDeadband.ctl" = cluster{"Name":string, "maxPositivePwm":i32, "minPositivePwm":i32, "centerPwm":i32, "maxNegativePwm":i32, "minNegativePwm":i32, "angularRange":u16}
  T19 = typedef "FPGA_DIOChannel.ctl" = enum8{"DIO 0", "DIO 1", "DIO 2", "DIO 3", "DIO 4", "DIO 5", "DIO 6", "DIO 7", "DIO 8", "DIO 9", "DIO MXP 0", "DIO MXP 1", "DIO MXP 2", "DIO MXP 3", "DIO MXP 4", "DIO MXP 5", "DIO MXP 6", "DIO MXP 7", "DIO MXP 8", "DIO MXP 9", "DIO MXP 10", "DIO MXP 11", "DIO MXP 12", "DIO MXP 13", "DIO MXP 14", "DIO MXP 15", "SPI Port CS1", "SPI Port CS2", "SPI Port CS3", "SPI Port MISO", "SPI Port MOSI", "Invalid"}
  T20 = typedef "ArmMotionProfileControl.ctl" = cluster{"ControlMutex":T21, "Trajectory Points":T22[], "CurrentIndex":u32}
  T21 = typedef "Semaphore RefNum" = refnum<k1>
  T22 = typedef "TrajectoryPoint.ctl" = cluster{"Position ":dbl, "Velocity ":dbl, "Time (ms)":T23, "Last Point":bool}
  T23 = typedef "CTRE_Phoenix_MotorControl_TrajectoryPointTimeDur.ctl" = i32
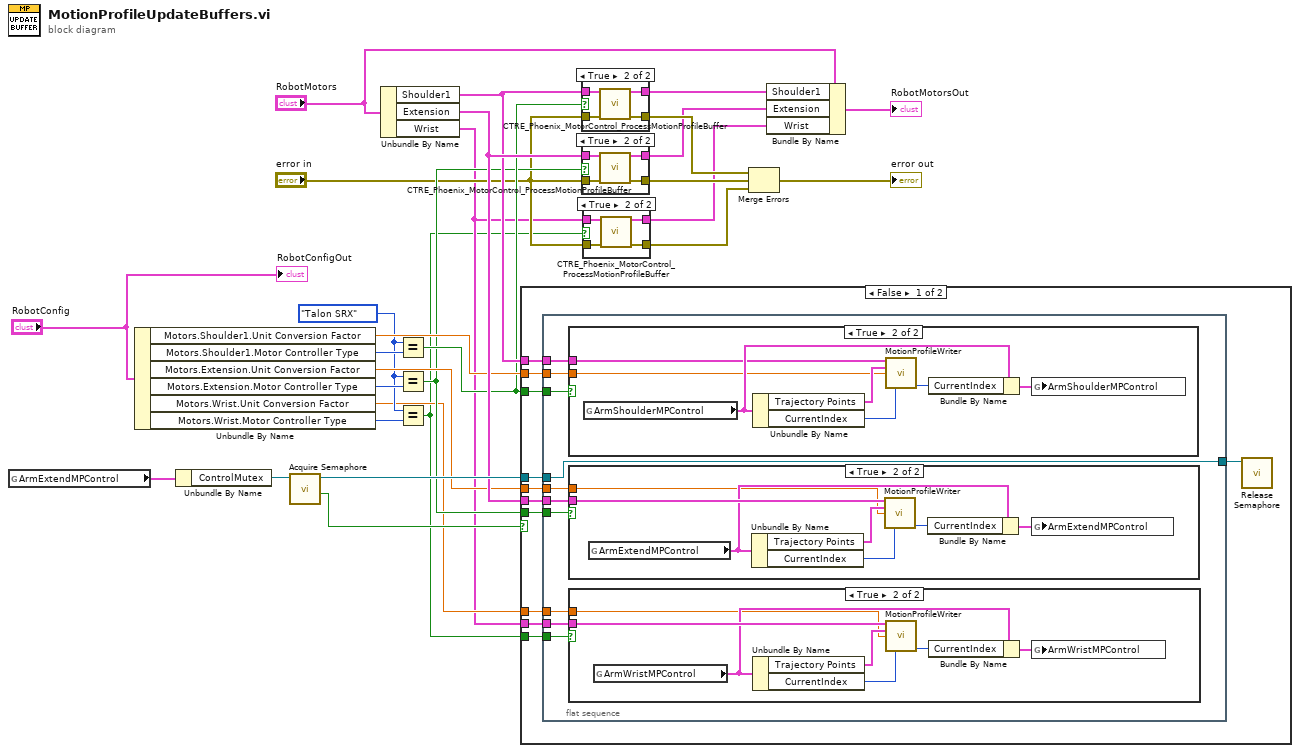
[diagram p0: block diagram]
diagram:
  w5 = Config_MotorCtrlType."Talon SRX" ("x")
  n1 = global read "MotionProfileControlData.vi" "ArmExtendMPControl"() -> (w19:T20)
  n2 = Unbundle By Name("RobotConfig") -> ("Motors.Shoulder1.Unit Conversion Factor"=w13:dbl, "Motors.Shoulder1.Motor Controller Type"=w12:T6, "Motors.Extension.Unit Conversion Factor"=w15:dbl, "Motors.Extension.Motor Controller Type"=w11:T6, "Motors.Wrist.Unit Conversion Factor"=w3:dbl, "Motors.Wrist.Motor Controller Type"=w4:T6)
  n3 = Unbundle By Name(w19) -> ("ControlMutex"=w20:T21)
  n4 = call <vilib>:"Acquire Semaphore.vi"("semaphore"=w20) -> ("timed out"=w17:bool, "semaphore out"=w21:T21)  [unwired: 4 in, 1 out]
  n5 = Unbundle By Name("RobotMotors") -> ("Shoulder1"=w14:T16, "Extension"=w18:T16, "Wrist"=w2:T16)
  n6 = Equal?(x=w5, y=w12) -> (x = y?=w10:bool)
  n7 = Equal?(x=w5, y=w11) -> (x = y?=w9:bool)
  n8 = Equal?(x=w5, y=w4) -> (x = y?=w1:bool)
  n9 = case shown="False" w17 {
    tunnel: w21 -> [w38 _]
    tunnel: w18 -> [w37 _]
    tunnel: w15 -> [w36 _]
    tunnel: w14 -> [w35 _]
    tunnel: w13 -> [w34 _]
    tunnel: w10 -> [w32 _]
    tunnel: w9 -> [w33 _]
    tunnel: w3 -> [w31 _]
    tunnel: w1 -> [w30 _]
    tunnel: w2 -> [w29 _]
    frame False {
      n10 = flat-sequence {
        tunnel: w37 -> [w49]
        tunnel: w38 -> [w45]
        tunnel: [w45] -> w39
        tunnel: w36 -> [w48]
        tunnel: w35 -> [w47]
        tunnel: w34 -> [w46]
        tunnel: w33 -> [w44]
        tunnel: w32 -> [w43]
        tunnel: w31 -> [w42]
        tunnel: w30 -> [w41]
        tunnel: w29 -> [w40]
        frame #0 {
          n11 = case shown="True" w43 {
            tunnel: w47 -> [_ w65]
            tunnel: w46 -> [_ w64]
            frame False {
            }
            frame True {
              n12 = global read "MotionProfileControlData.vi" "ArmShoulderMPControl"() -> (w68:T20)
              n13 = Unbundle By Name(w68) -> ("Trajectory Points"=w66:T22[], "CurrentIndex"=w67:u32)
              n14 = call "MotionProfileWriter.vi"("PhoenixMotorControlDevRef"=w65, "Trajectory Points"=w66, "Sensor unit conversion"=w64, "startIndex"=w67) -> ("endIndex"=w69:i32)  [unwired: 10 in, 1 out]
              n15 = Bundle By Name(cluster=w68, "CurrentIndex"=w69) -> (w70:T20)
              n16 = global write "MotionProfileControlData.vi" "ArmShoulderMPControl"(w70) -> ()
            }
          }
          n17 = case shown="True" w44 {
            tunnel: w49 -> [_ w63]
            tunnel: w48 -> [_ w57]
            frame False {
            }
            frame True {
              n18 = global read "MotionProfileControlData.vi" "ArmExtendMPControl"() -> (w60:T20)
              n19 = Unbundle By Name(w60) -> ("Trajectory Points"=w62:T22[], "CurrentIndex"=w61:u32)
              n20 = call "MotionProfileWriter.vi"("PhoenixMotorControlDevRef"=w63, "Trajectory Points"=w62, "Sensor unit conversion"=w57, "startIndex"=w61) -> ("endIndex"=w59:i32)  [unwired: 10 in, 1 out]
              n21 = Bundle By Name(cluster=w60, "CurrentIndex"=w59) -> (w58:T20)
              n22 = global write "MotionProfileControlData.vi" "ArmExtendMPControl"(w58) -> ()
            }
          }
          n23 = case shown="True" w41 {
            tunnel: w40 -> [_ w56]
            tunnel: w42 -> [_ w50]
            frame False {
            }
            frame True {
              n24 = global read "MotionProfileControlData.vi" "ArmWristMPControl"() -> (w53:T20)
              n25 = Unbundle By Name(w53) -> ("Trajectory Points"=w55:T22[], "CurrentIndex"=w54:u32)
              n26 = call "MotionProfileWriter.vi"("PhoenixMotorControlDevRef"=w56, "Trajectory Points"=w55, "Sensor unit conversion"=w50, "startIndex"=w54) -> ("endIndex"=w52:i32)  [unwired: 10 in, 1 out]
              n27 = Bundle By Name(cluster=w53, "CurrentIndex"=w52) -> (w51:T20)
              n28 = global write "MotionProfileControlData.vi" "ArmWristMPControl"(w51) -> ()
            }
          }
        }
      }
      n29 = call <vilib>:"Release Semaphore.vi"("semaphore"=w39) -> ()  [unwired: 5 in, 2 out]
    }
    frame True {
    }
  }
  n30 = case shown="True" w10 {
    tunnel: "error in" -> [w71 w76]
    tunnel: [w71 w75] -> w28
    tunnel: [w72 w74] -> w23
    tunnel: w14 -> [w72 w73]
    frame False {
    }
    frame True {
      n31 = call <vilib>:"CTRE_Phoenix_MotorControl_ProcessMotionProfileBuffer.vi"("PhoenixMotorControlDevRef"=w73, "error in"=w76) -> ("PhoenixMotorControlDevRef"=w74:T16, "error out"=w75:errorcluster)  [unwired: 12 in]
    }
  }
  n32 = case shown="True" w9 {
    tunnel: "error in" -> [w77 w82]
    tunnel: [w77 w81] -> w27
    tunnel: [w78 w80] -> w22
    tunnel: w18 -> [w78 w79]
    frame False {
    }
    frame True {
      n33 = call <vilib>:"CTRE_Phoenix_MotorControl_ProcessMotionProfileBuffer.vi"("PhoenixMotorControlDevRef"=w79, "error in"=w82) -> ("PhoenixMotorControlDevRef"=w80:T16, "error out"=w81:errorcluster)  [unwired: 12 in]
    }
  }
  n34 = case shown="True" w1 {
    tunnel: "error in" -> [w83 w88]
    tunnel: [w83 w87] -> w7
    tunnel: [w84 w86] -> w6
    tunnel: w2 -> [w84 w85]
    frame False {
    }
    frame True {
      n35 = call <vilib>:"CTRE_Phoenix_MotorControl_ProcessMotionProfileBuffer.vi"("PhoenixMotorControlDevRef"=w85, "error in"=w88) -> ("PhoenixMotorControlDevRef"=w86:T16, "error out"=w87:errorcluster)  [unwired: 12 in]
    }
  }
  n36 = Merge Errors(w28, w27, w7) -> (→"error out":errorcluster)
  n37 = Bundle By Name(cluster="RobotMotors", "Shoulder1"=w23, "Extension"=w22, "Wrist"=w6) -> (→"RobotMotorsOut":T15)
  "RobotConfigOut" <- "RobotConfig"
